vi "TIC Query Command.vi"(8 "error in (no error)":errorcluster, 10 "Command String":string, 11 "VISA Resource Name":refnum<visa-resource-name>) -> (0 "error out":errorcluster {"code" format="%.0x"}, 2 "Truncated Respose":string, 3 "VISA session (Dup)":refnum<visa-resource-name>)   [LabVIEW 2018]
doc: "Sends a command or query to the TIC, and then reads back and parses the response."
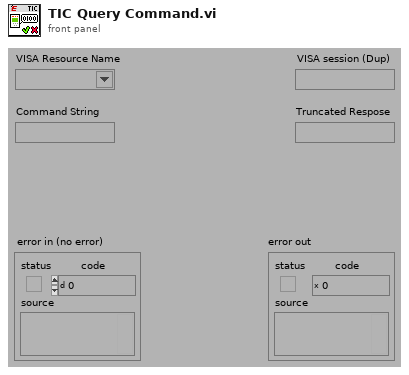
[diagram p1: front panel]
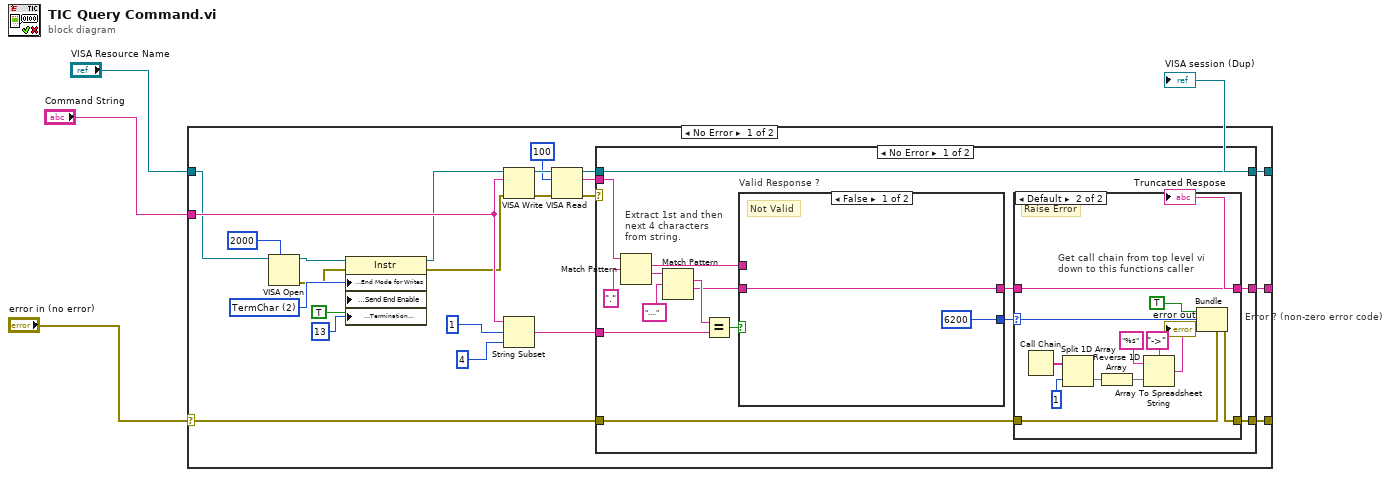
[diagram p0: block diagram]
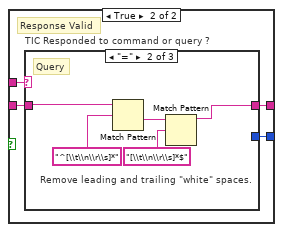
[diagram p3: hidden frame]
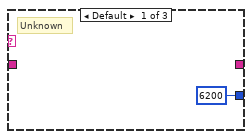
[diagram p4: hidden frame]
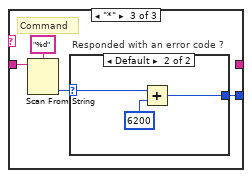
[diagram p5: hidden frame]
diagram:
  n1 = case shown="No Error" "error in (no error)" {
    selector: "error in (no error)" -> [w21 w80]
    tunnel: "VISA Resource Name" -> [w9 w81]
    tunnel: [w25 w80] -> w5
    tunnel: [w23 w81] -> w4
    tunnel: "Command String" -> [w20 _]
    tunnel: [w16 _] -> w1
    frame No Error {
      w14 = u16 2 items=["None", "Last Bit", "TermChar", "Break"] ("Serial Settings:End Mode for Writes")
      n2 = VISA Open(timeout (0)=u32 2000 ("VISA Open timeout (0)"), VISA resource name=w9) -> (VISA resource name=w11:refnum<visa-resource-name>, error out=w10:errorcluster)  [unwired: 3 in]
      n3 = property class="Instr"(reference=w11, error in=w10, "Serial Settings:End Mode for Writes"=w14, "Message Based Settings:Send End Enable"=TRUE, "Message Based Settings:Termination Character"=u8 13) -> (reference out=w8:refnum<visa-resource-name>, error out=w7:errorcluster)
      n4 = VISA Write(VISA resource name=w8, write buffer=w20, error in (no error)=w7) -> (VISA resource name out=w29:refnum<visa-resource-name>, error out=w28:errorcluster)  [unwired: 1 out]
      n5 = String Subset(string=w20, offset (0)=1, length (rest)=4 ("length (rest)")) -> (substring=w17:string)
      n6 = VISA Read(VISA resource name=w29, byte count=u32 100 ("byte count (0)"), error in (no error)=w28) -> (VISA resource name out=w24:refnum<visa-resource-name>, read buffer=w26:string, error out=w22:errorcluster)  [unwired: 1 out]
      n7 = case shown="No Error" w22 {
        selector: w22 -> [_ w78]
        tunnel: w26 -> [w42 _]
        tunnel: w21 -> [w32 _]
        tunnel: [w31 w78] -> w25
        tunnel: w24 -> [w44 w79]
        tunnel: [w44 w79] -> w23
        tunnel: w17 -> [w39 _]
        tunnel: [w30 _] -> w16
        frame No Error {
          # "Extract 1st and then\nnext 4 characters\nfrom string."
          n8 = Match Pattern(string=w42, regular expression=".") -> (match substring=w37:string, after substring=w41:string)  [unwired: 1 in, 2 out]
          n9 = Match Pattern(string=w41, regular expression="....") -> (match substring=w38:string, after substring=w36:string)  [unwired: 1 in, 2 out]
          n10 = Equal?(x=w38, y=w39) -> (x = y?=w35:bool)
          n11 = case "Valid Response ?" shown="False" w35 {
            tunnel: w37 -> [_ w64]
            tunnel: w36 -> [w60 w63]
            tunnel: [w60 w62] -> w33
            tunnel: [6200 ("code") w61] -> w34
            frame False {
              # "Not Valid"
            }
            frame True {
              # "Response Valid"
              n12 = case "TIC Responded to command or query ?" shown="\"=\"" w64 {
                tunnel: w63 -> [_ w67 w73]
                tunnel: [_ w66 _] -> w62
                tunnel: [6200 _ w71] -> w61
                frame Default {
                  # "Unknown"
                }
                frame "=" {
                  # "Remove leading and trailing \"white\" spaces."
                  # "Query"
                  n13 = Match Pattern(string=w67, regular expression="^[\\t\\n\\r\\s]*") -> (after substring=w70:string)  [unwired: 1 in, 3 out]
                  n14 = Match Pattern(string=w70, regular expression="[\\t\\n\\r\\s]*$") -> (before substring=w66:string)  [unwired: 1 in, 3 out]
                }
                frame "*" {
                  # "Command"
                  n15 = Scan From String(format string="%d", input string=w73) -> (output 1=w72:i32)  [unwired: 3 in, 3 out]
                  n16 = case "Responded with an error code ?" shown="Default" w72 {
                    selector: w72 -> [_ w76]
                    tunnel: [_ w75] -> w71
                    frame 0 {
                    }
                    frame Default {
                      n17 = Add(x=w76, y=6200) -> (x+y=w75:i32)
                    }
                  }
                }
              }
            }
          }
          n18 = case "Error ? (non-zero error code)" shown="Default" w34 {
            selector: w34 -> [_ w50]
            tunnel: w33 -> [w46 w47]
            tunnel: w32 -> [w45 w49]
            tunnel: [w45 w48] -> w31
            tunnel: [w46 w47] -> w30
            frame 0 {
              # "No Error"
            }
            frame Default {
              # "Get call chain from top level vi\ndown to this functions caller"
              # "Raise Error"
              n19 = Call Chain() -> (call chain=w54:string[])
              n20 = Split 1D Array(array=w54, index=1) -> (second subarray=w56:string[])  [unwired: 1 out]
              n21 = Reverse 1D Array(array=w56) -> (reversed array=w57:string[])
              n22 = Array To Spreadsheet String(delimiter (Tab)="->", array=w57, 3:"%s" ("format string")) -> (spreadsheet string=w51:string)
              n23 = Bundle(cluster=w49, "status"=TRUE, "code"=w50, "source"=w51) -> (w48:errorcluster)
            }
          }
        }
        frame Error {
        }
      }
    }
    frame Error {
    }
  }
  "error out" <- w5
  "Truncated Respose" <- w1
  "VISA session (Dup)" <- w4
